vi "ResizeToBiggestDecoration.vi"(8 "error in (no error)":errorcluster, 10 "Resize By":T1(ring), 11 "VI in":refnum<vi>) -> (0 "error out":errorcluster)   [LabVIEW 2023, in "FolloWin.lvclass"]
doc: "This VI sets VI referenced by VI in to its front panel bounds to biggest decoration by area"
uses:
  FolloWin.lvclass
  FolloWin.lvclass/FolloWin.ctl
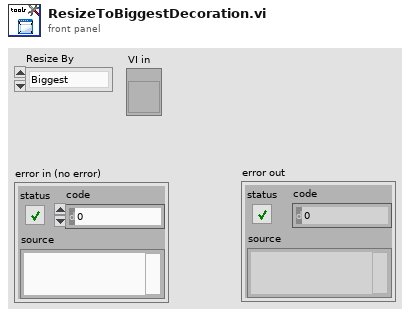
[diagram p1: front panel]
types:
  T1 = enum16{"Biggest", "Rightmost", "Leftmost", "Topmost", "Bottommost"}
  T2 = typedef "LVBoundsTypeDef.ctl" = cluster{"Width":u32, "Height":u32}
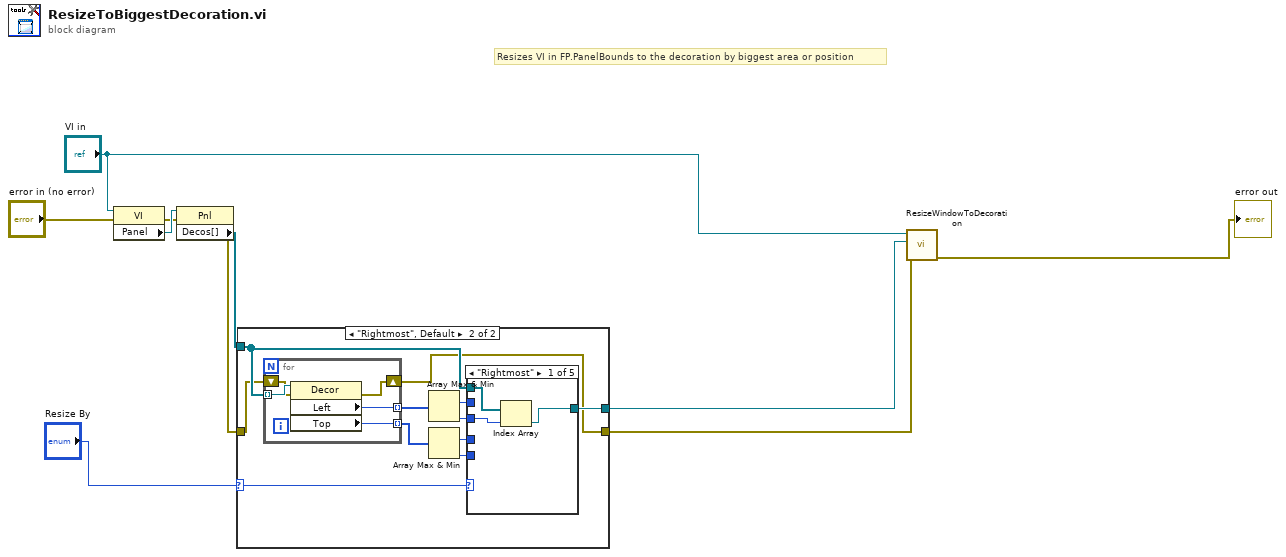
[diagram p0: block diagram]
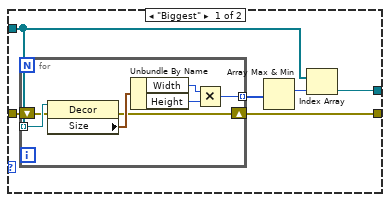
[diagram p2: hidden frame]
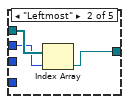
[diagram p3: hidden frame]
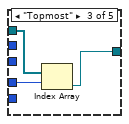
[diagram p4: hidden frame]
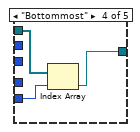
[diagram p5: hidden frame]
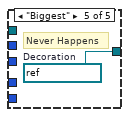
[diagram p6: hidden frame]
diagram:
  # "Resizes VI in FP.PanelBounds to the decoration by biggest area or position"
  n1 = property on="Property Node" class="VI"(reference="VI in", error in="error in (no error)") -> (error out=w6:errorcluster, "Panel"=w8:refnum<vi>)  [unwired: 1 out]
  n2 = property on="Property Node" class="Pnl"(reference=w8, error in=w6) -> (error out=w5:errorcluster, "Decos[]"=w7:refnum<vi>[])  [unwired: 1 out]
  n3 = case shown="\"Rightmost\", Default" "Resize By" {
    selector: "Resize By" -> [_ w34]
    tunnel: [w16 w29] -> w9
    tunnel: w7 -> [w15 w31]
    tunnel: w5 -> [w12 w25]
    tunnel: [w11 w24] -> w4
    frame "Biggest" {
      n4 = for {
        tunnel: w15 -> [w23] mode=indexing
        tunnel: [w19] -> w13 mode=indexing
        shift-right: [w17] -> w11
        shift-left: w12 -> [w18]
        n5 = property on="Property Node" class="Decor"(reference=w23, error in=w18) -> (error out=w17:errorcluster, "Size"=w22:T2)  [unwired: 1 out]
        n6 = Unbundle By Name(w22) -> ("Width"=w20:u32, "Height"=w21:u32)
        n7 = Multiply(x=w20, y=w21) -> (x*y=w19:u32)
      }
      n8 = Array Max & Min(array=w13) -> (max index (indices)=w14:i32)  [unwired: 3 out]
      n9 = Index Array(array=w15, index=w14) -> (element=w16:refnum<vi>)
    }
    frame "Rightmost", Default {
      n10 = for {
        tunnel: w31 -> [w39] mode=indexing
        tunnel: [w38] -> w33 mode=indexing
        tunnel: [w37] -> w32 mode=indexing
        shift-right: [w35] -> w24
        shift-left: w25 -> [w36]
        n11 = property class="Decor"(reference=w39, error in=w36) -> (error out=w35:errorcluster, "Left"=w38:i32, "Top"=w37:i32)  [unwired: 1 out]
      }
      n12 = Array Max & Min(array=w33) -> (max index (indices)=w30:i32, min index (indices)=w28:i32)  [unwired: 2 out]
      n13 = Array Max & Min(array=w32) -> (max index (indices)=w27:i32, min index (indices)=w26:i32)  [unwired: 2 out]
      n14 = case shown="\"Rightmost\"" w34 {
        tunnel: w31 -> [w42 w45 w48 w51 _]
        tunnel: w30 -> [_ w44 _ _ _]
        tunnel: [w41 w43 w47 w50 w52] -> w29
        tunnel: w28 -> [w40 _ _ _ _]
        tunnel: w27 -> [_ _ w46 _ _]
        tunnel: w26 -> [_ _ _ w49 _]
        frame "Rightmost" {
          n15 = Index Array(array=w42, index=w40) -> (element=w41:refnum<vi>)
        }
        frame "Leftmost" {
          n16 = Index Array(array=w45, index=w44) -> (element=w43:refnum<vi>)
        }
        frame "Topmost" {
          n17 = Index Array(array=w48, index=w46) -> (element=w47:refnum<vi>)
        }
        frame "Bottommost" {
          n18 = Index Array(array=w51, index=w49) -> (element=w50:refnum<vi>)
        }
        frame "Biggest" {
          w52 = refnum<vi> refnum  # Decoration
          # "Never Happens"
        }
      }
    }
  }
  n19 = call "ResizeWindowToDecoration.vi"("error in (no error)"=w4, "Decor Refnum"=w9, "VI in"="VI in") -> ("error out"=→"error out":errorcluster)  [unwired: 8 in]
